vi "SSI_Query ID.vi"(6 "Timeout":u32=1000, 7 "Number of bytes":u32=4096, 8 "Error in (no error)":errorcluster caption="error out（no error）", 9 "Remote Mode":u16(ring) items=["USB", "RS232", "GPIB", "Ethernet"], 10 "Connection ID in":refnum<k5>, 11 "VISA resource name":refnum<visa-resource-name>) -> (0 "Error out":errorcluster caption="error out", 1 "Read Buffer":string, 2 "Connection ID out":refnum<k5>, 3 "VISA resource  out":refnum<visa-resource-name>)   [LabVIEW 2019]
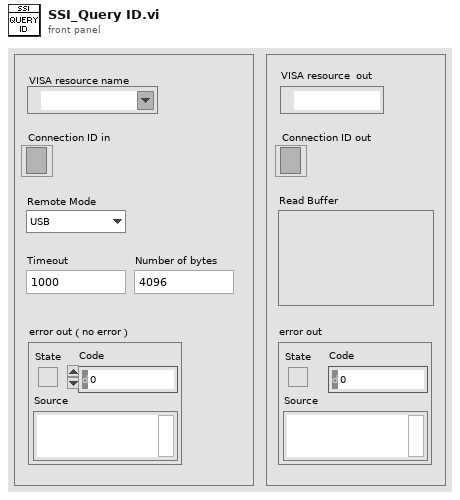
[diagram p1: front panel]
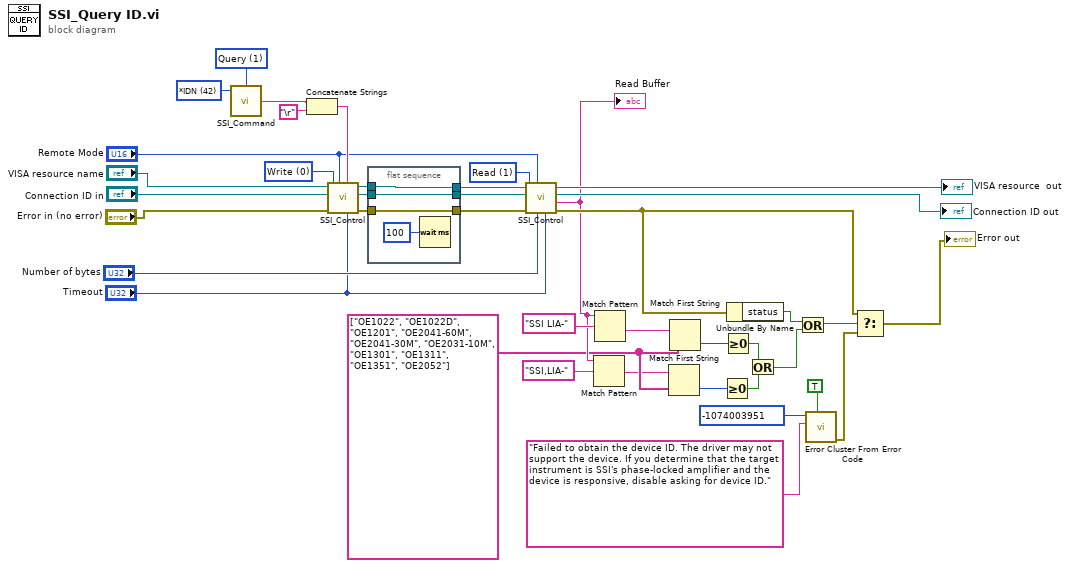
[diagram p0: block diagram]
diagram:
  w9 = u16 42 items=["ISRC", "IGND", "ICPL", "ILIN", "PHAS", "FMOD", "RSLP", "FREQ", "SWPT", "SLLM", "SULM", "SSLL", "SSLG", "STLM", "SWRM", "IRNG", "SENS", "RMOD", "OFLT", "OFSL", "SYNC", "DMOD", "HARM", "DARB", "SWVT", "SLVL", "SVLL", "SVUL", "SVSL", "SVSG", "SVTM", "SVRM", "RALL", "SNAP", "OUTP", "OAUX", "COUT", "CAUX", "COFP", "CEXP", "FPOP", "OEXP", "*IDN", "*RST", "OVLD", "INOV", "GNOV", "*PLL", "SSET", "RSET", "AGAN", "APHS", "ARSV", "ASCL", "EQCD", "EQCS", "SPED", "SRAT", "SLEN", "SSLE", "STRG", "SPRM", "STRD", "PAUS", "REST", "SPTS", "TRCA", "TEMP", "RSTU", "IHNZ", "DEQU", "SADD", "ARNG", "CSPE", "ISRCD", "IGNDD", "ICPLD", "ILIND", "PHASD", "FMODD", "RSLPD", "FREQD", "SWPTD", "SLLMD", "SULMD", "SSLLD", "SSLGD", "STLMD", "SWRMD", "SENSD", "RMODD", "OFLTD", "OFSLD", "SYNCD", "HARMD", "EQCDD", "EQCSD", "SNAPD", "OUTPD", "SWVTD", "SLVLD", "SVLLD", "SVULD", "SVSLD", "SVSGD", "SVTMD", "SVRMD", "SVDCD", "ARSVD", "AGAND", "APHSD", "ASCLD", "FPOPD", "CAUXD", "OEXPD", "SPEDD", "SRATD", "SLEND", "SSLED", "STRGD", "SPRMD", "STRDD", "PAUSD", "RESTD", "SPTSD", "TRCAD", "*IDND", "*RSTD", "INOVD", "GNOVD", "*PLLD", "SSETD", "RSETD", "RALLD"] ("Command Type")
  w20 = u16 1 items=["Set", "Query"] ("Opera")
  w27 = u16 1 items=["Write", "Read"] ("Opera")
  w28 = u16 0 items=["Write", "Read"] ("Opera")
  w4 = string[] ["OE1022", "OE1022D", "OE1201", "OE2041-60M", "OE2041-30M", "OE2031-10M", "OE1301", "OE1311", "OE1351", "OE2052"] ("string array")
  n1 = call "SSI_Command.vi"("Opera"=w20, "Command Type"=w9) -> ("Output string"=w31:string)  [unwired: 2 in]
  n2 = Concatenate Strings(w31, "\r") -> (w30:string)
  n3 = call "SSI_Control.vi"("Tineout"="Timeout", "Write Buffer"=w30, "Remote Mode"="Remote Mode", "Error in (no error)"="Error in (no error)", "Control"=w28, "Connection ID in"="Connection ID in", "VISA resource name"="VISA resource name") -> ("Error out"=w16:errorcluster, "Connection ID out"=w17:refnum<k5>, "VISA resource  out"=w18:refnum<visa-resource-name>)  [unwired: 1 in, 1 out]
  n4 = flat-sequence {
    tunnel: w18 -> [w41]
    tunnel: w17 -> [w42]
    tunnel: w16 -> [w43]
    tunnel: [w43] -> w14
    tunnel: [w42] -> w13
    tunnel: [w41] -> _
    tunnel: [w41] -> w15
    frame #0 {
      n5 = Wait (ms)(milliseconds to wait=u32 100 ("等待时间（毫秒）")) -> ()  [unwired: 1 out]
    }
  }
  n6 = call "SSI_Control.vi"("Tineout"="Timeout", "Number of bytes"="Number of bytes", "Remote Mode"="Remote Mode", "Error in (no error)"=w14, "Control"=w27, "Connection ID in"=w13, "VISA resource name"=w15) -> ("Error out"=w25:errorcluster, "Read Buffer"=w6:string, "Connection ID out"=→"Connection ID out":refnum<k5>, "VISA resource  out"=→"VISA resource  out":refnum<visa-resource-name>)  [unwired: 1 in]
  "Read Buffer" <- w6
  n7 = Match Pattern(string=w6, regular expression="SSI,LIA-" ("字符串")) -> (after substring=w3:string)  [unwired: 1 in, 3 out]
  n8 = Match Pattern(string=w6, regular expression="SSI LIA-" ("正则表达式")) -> (after substring=w39:string)  [unwired: 1 in, 3 out]
  n9 = Match First String(2:w4, 3:w3) -> (0:w7:i32)  [unwired: 1 out]
  n10 = Match First String(2:w4, 3:w39) -> (0:w40:i32)  [unwired: 1 out]
  n11 = Greater Or Equal To 0?(x=w7) -> (x >= 0?=w2:bool)
  n12 = Greater Or Equal To 0?(x=w40) -> (x >= 0?=w8:bool)
  n13 = Unbundle By Name(w25) -> ("status"=w38:bool)
  n14 = Or(x=w8, y=w2) -> (x .or. y?=w1:bool)
  n15 = Or(x=w38, y=w1) -> (x .or. y?=w37:bool)
  n16 = call <vilib>:"Error Cluster From Error Code.vi"("show call chain? (False)"=TRUE, "error message (\"\")"="Failed to obtain the device ID. The driver may not support the device. If you determine that the target instrument is SSI's phase-locked amplifier and the device is responsive, disable asking for device ID." ("Source (VI Name)"), "error code (0)"=-1074003951 ("Code")) -> ("error out"=w33:errorcluster)  [unwired: 1 in, 5 out]
  n17 = Select(t=w25, s=w37, f=w33) -> (s? t:f=→"Error out":errorcluster)
